vi "RelativeResize.vi"(5 "Image Type":T1=4 items=["Grayscale (U8)", "Grayscale (I16)", "Grayscale (SGL)", "Complex (CSG)", "RGB (U32)", "HSL (U32)", "RGB (U64)", "Grayscale (U16)"], 6 "error in":errorcluster, 7 "Desired X Resolution":i32=640, 8 "Image Dst":T2, 9 "Image":T2) -> (0 "error out":errorcluster, 1 "Y Resolution":i32, 2 "X Resolution":i32, 3 "Image Dst Out":T2)   [LabVIEW 2009]
uses:
  <vilib>/vision/Image Controls.llb/IMAQ Image.ctl
  <vilib>/vision/NI_Vision_Development_Module.lvlib
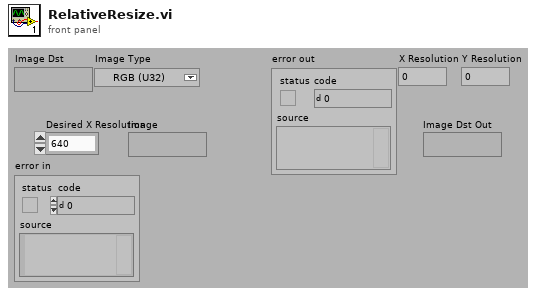
[diagram p1: front panel]
types:
  T1 = typedef "Image Type" = u32
  T2 = typedef "IMAQ Image.ctl" = refnum<image>
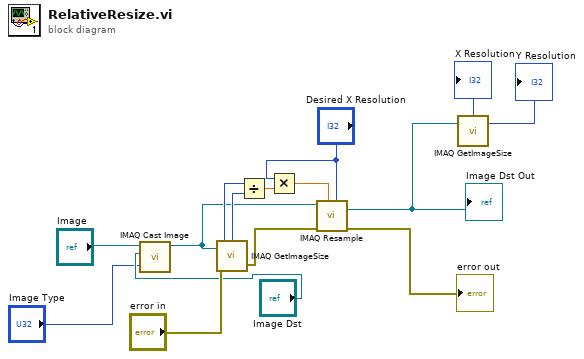
[diagram p0: block diagram]
diagram:
  n1 = call "IMAQ Cast Image"("Image Type"="Image Type", "Image Dst"="Image Dst", "Image Src"="Image") -> ("Image Dst Out"=w4:T2)  [unwired: 7 in, 1 out]
  n2 = call "IMAQ GetImageSize"("Image"=w4, "error in (no error)"="error in") -> ("Y Resolution"=w15:i32, "X Resolution"=w13:i32, "error out"=w11:errorcluster)  [unwired: 2 in]
  n3 = Divide(x=w15, y=w13) -> (x/y=w12:dbl)
  n4 = Multiply(x="Desired X Resolution", y=w12) -> (x*y=w14:dbl)
  n5 = call "IMAQ Resample"("X Resolution"="Desired X Resolution", "Y Resolution"=w14, "error in (no error)"=w11, "Image Src"=w4) -> ("error out"=→"error out":errorcluster, "Image Dst Out"=w8:T2)  [unwired: 6 in]
  "Image Dst Out" <- w8
  n6 = call "IMAQ GetImageSize"("Image"=w8) -> ("Y Resolution"=→"Y Resolution":i32, "X Resolution"=→"X Resolution":i32)  [unwired: 3 in, 1 out]
